vi "Initialize.vi"() -> (3 "asset utilization":refnum<class "NI SystemLink Asset Utilization.lvclass">)   [LabVIEW 2019]
uses:
  <vilib>/Skyline/AssetManagement/NI SystemLink Asset Utilization.lvclass
  <vilib>/Skyline/AssetManagement/Start Utilization (All).vi
  <vilib>/Skyline/AssetManagement/Start Utilization (Single).vi
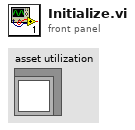
[diagram p1: front panel]
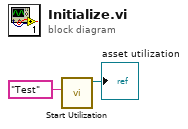
[diagram p0: block diagram]
diagram:
  n1 = call-poly <vilib>:"Start Utilization.vi"("utilization category"="Test") -> ("asset utilization"=→"asset utilization":refnum<class "NI SystemLink Asset Utilization.lvclass">)  [unwired: 9 in, 1 out]
